vi "Get ActiveResultsSpace.vi"(8 "error in (no error)":errorcluster, 11 "niDTS BT INSTR TX in":refnum<class "niDTS BT INSTR TX.lvclass">) -> (0 "error out":errorcluster, 2 "ActiveResultsSpace":u8=1 min=1 step=1, 3 "niDTS BT INSTR TX out":refnum<class "niDTS BT INSTR TX.lvclass">)   [LabVIEW 2015, in "niDTS BT.lvlib" / "niDTS BT INSTR TX.lvclass"]
uses:
  niDTS BT INSTR TX.lvclass
  niDTS BT INSTR TX.lvclass/niDTS BT INSTR TX.ctl
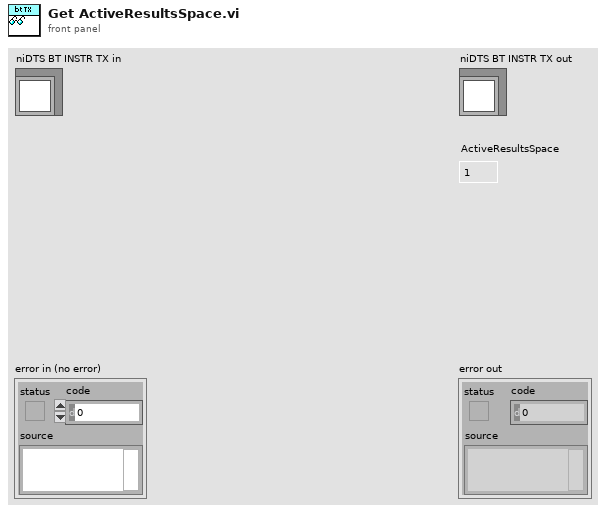
[diagram p1: front panel]
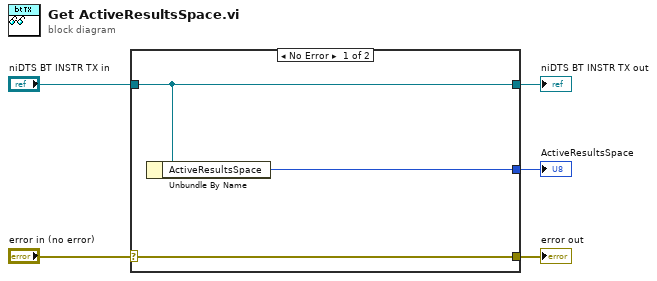
[diagram p0: block diagram]
diagram:
  n1 = case shown="No Error" "error in (no error)" {
    selector: "error in (no error)" -> [w8 w9]
    tunnel: [w8 w9] -> w4
    tunnel: [w7 w10] -> w2
    tunnel: "niDTS BT INSTR TX in" -> [w7 w10]
    tunnel: [w6 _] -> w1
    frame No Error {
      n2 = Unbundle By Name(w7) -> ("ActiveResultsSpace"=w6:u8)
    }
    frame Error {
    }
  }
  "error out" <- w4
  "niDTS BT INSTR TX out" <- w2
  "ActiveResultsSpace" <- w1
